vi "Close.vi"(8 "error in (no error)":errorcluster, 11 "DO (N Samples) Ref In":T1) -> (0 "error out":errorcluster)   [LabVIEW 2021, in "DO Block.lvlib"]
doc: "Closes the reference to one or more digital output channels, sets the logic levels of the digital output channels to low, and disables digital output channels."
uses:
  <vilib>/myRIO/Instrument Drivers/Onboard IO/DO Block/DO Block.lvlib
  <vilib>/myRIO/Instrument Drivers/Onboard IO/DO Block/typedefs/DO Block Reference.ctl
  <vilib>/myRIO/Common/Instrument Driver Framework/Utilities/typedefs/myRIO Generic Hardware Reference.ctl
  <vilib>/myRIO/Common/Instrument Driver Framework/Utilities/typedefs/Hardware Version Enum.ctl
  <vilib>/myRIO/Common/Instrument Driver Framework/Utilities/typedefs/myRIO v1.0 Reference.ctl
  <vilib>/myRIO/Common/Instrument Driver Framework/Utilities/typedefs/Generic FPGA Reference.ctl
  <vilib>/myRIO/Common/Instrument Driver Framework/myRIO v1.0/DO Block/typedefs/DO Block Channels List.ctl
  <vilib>/myRIO/Common/Instrument Driver Framework/myRIO v1.0/DO Block/typedefs/DO Block Channels Enum.ctl
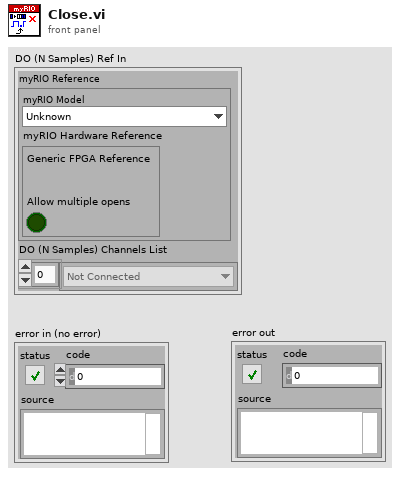
[diagram p1: front panel]
types:
  T1 = typedef "DO Block.lvlib/DO Block Reference.ctl" = cluster{"myRIO Reference":T2, "DO (N Samples) Channels List":T6}
  T2 = typedef "myRIO Generic Hardware Reference.ctl" = cluster{"myRIO Model":T3, "myRIO Hardware Reference":T4}
  T3 = typedef "Hardware Version Enum.ctl" = enum16{"Unknown", "myRIO-1900", "myRIO-1950", "roboRIO", "NI ELVIS RIO CM", "ELVIS III"}
  T4 = typedef "myRIO v1.0 Reference.ctl" = cluster{"Generic FPGA Reference":T5, "Allow multiple opens":bool}
  T5 = typedef "Generic FPGA Reference.ctl" = refnum<k20>
  T6 = typedef "DO Block Channels List.ctl" = T7[]
  T7 = typedef "DO Block Channels Enum.ctl" = enum16{"Not Connected", "A/DO0 (N Samples)", "A/DO1 (N Samples)", "A/DO2 (N Samples)", "A/DO3 (N Samples)", "A/DO4 (N Samples)", "A/DO5 (N Samples)", "A/DO6 (N Samples)", "A/DO7 (N Samples)", "A/DO8 (N Samples)", "A/DO9 (N Samples)", "A/DO10 (N Samples)", "A/DO11 (N Samples)", "A/DO12 (N Samples)", "A/DO13 (N Samples)", "A/DO14 (N Samples)", "A/DO15 (N Samples)", "A/DO16 (N Samples)", "A/DO17 (N Samples)", "A/DO18 (N Samples)", "A/DO19 (N Samples)", "B/DO0 (N Samples)", "B/DO1 (N Samples)", "B/DO2 (N Samples)", "B/DO3 (N Samples)", "B/DO4 (N Samples)", "B/DO5 (N Samples)", "B/DO6 (N Samples)", "B/DO7 (N Samples)", "B/DO8 (N Samples)", "B/DO9 (N Samples)", "B/DO10 (N Samples)", "B/DO11 (N Samples)", "B/DO12 (N Samples)", "B/DO13 (N Samples)", "B/DO14 (N Samples)", "B/DO15 (N Samples)", "B/DO16 (N Samples)", "B/DO17 (N Samples)", "B/DO18 (N Samples)", "B/DO19 (N Samples)"}
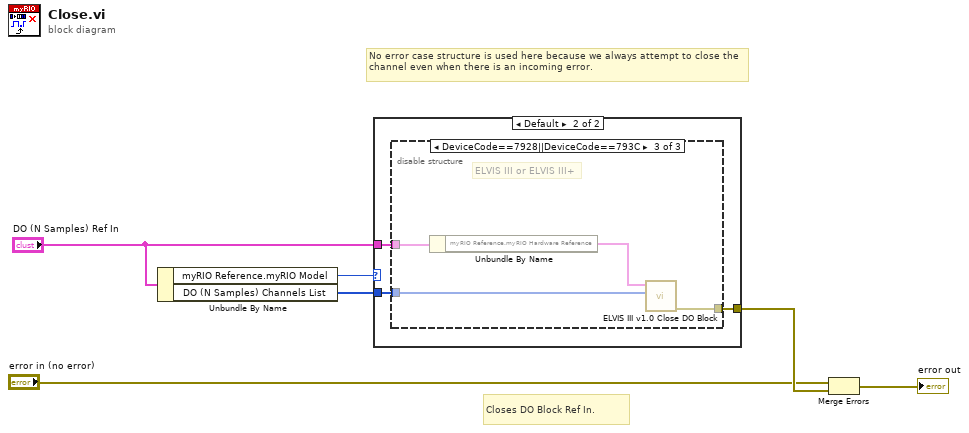
[diagram p0: block diagram]
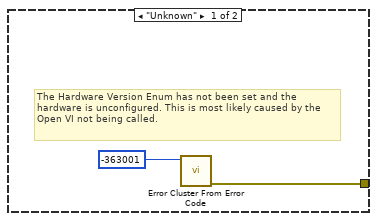
[diagram p2: hidden frame]
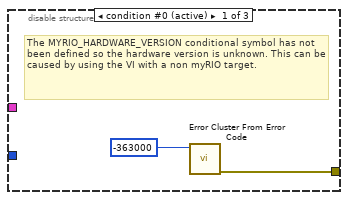
[diagram p3: hidden frame]
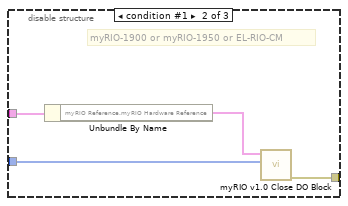
[diagram p4: hidden frame]
diagram:
  # "Closes DO Block Ref In."
  # "No error case structure is used here because we always attempt to close the channel even when there is an incoming error."
  n1 = Unbundle By Name("DO (N Samples) Ref In") -> ("myRIO Reference.myRIO Model"=w5:T3, "DO (N Samples) Channels List"=w6:T6)
  n2 = case shown="Default" w5 {
    tunnel: "DO (N Samples) Ref In" -> [_ w11]
    tunnel: [w7 w10] -> w4
    tunnel: w6 -> [_ w9]
    frame "Unknown" {
      # "The Hardware Version Enum has not been set and the hardware is unconfigured. This is most likely caused by the Open VI not being called."
      n3 = call <vilib>:"Error Cluster From Error Code.vi"("error code (0)"=-363001) -> ("error out"=w7:errorcluster)  [unwired: 8 in]
    }
    frame Default {
      n4 = disable-structure shown="DeviceCode==7928||DeviceCode==793C" {
        disable-tunnel: w11 -> [_ w17 w20]
        disable-tunnel: [w12 w16 w18] -> w10
        disable-tunnel: w9 -> [_ w15 w19]
        frame condition #0 (active) {
          # "The MYRIO_HARDWARE_VERSION conditional symbol has not been defined so the hardware version is unknown. This can be caused by using the VI with a non myRIO target."
          n5 = call <vilib>:"Error Cluster From Error Code.vi"("error code (0)"=-363000) -> ("error out"=w12:errorcluster)  [unwired: 8 in]
        }
        frame condition #1 {
          # "myRIO-1900 or myRIO-1950 or EL-RIO-CM"
          n6 = Unbundle By Name(w17) -> ("myRIO Reference.myRIO Hardware Reference"=w14:T4)
          n7 = call <vilib>:"myRIO v1.0 Close DO Block.vi"("DO (N Samples) Channel List"=w15, "myRIO Ref In"=w14) -> ("error out"=w16:errorcluster)  [unwired: 9 in]
        }
        frame condition #2 {
          # "ELVIS III or ELVIS III+"
          n8 = Unbundle By Name(w20) -> ("myRIO Reference.myRIO Hardware Reference"=w21:T4)
          n9 = call <vilib>:"ELVIS III v1.0 Close DO Block.vi"("DO (N Samples) Channel List"=w19, "myRIO Ref In"=w21) -> ("error out"=w18:errorcluster)  [unwired: 9 in]
        }
      }
    }
  }
  n10 = Merge Errors("error in (no error)", w4) -> (→"error out":errorcluster)
